vi "nav_test.vi"() -> ()   [LabVIEW 2009]
uses:
  Seagle_2010_v2.0 - rewrite.llb/GPGLL data.ctl
  Seagle_2010_v2.0 - rewrite.llb/GPVTG data.ctl
  Seagle_2010_v2.0 - rewrite.llb/GPGSA data.ctl
  Seagle_2010_v2.0 - rewrite.llb/GPGSV data.ctl
  Seagle_2010_v2.0 - rewrite.llb/GPRMC data.ctl
  Seagle_2010_v2.0 - rewrite.llb/GPSINS output.ctl
  <vilib>/Instr/_visa.llb/VISA Configure Serial Port (Instr).vi
  Seagle_2010_v2.0 - rewrite.llb/GPS_Data_Global_Var.vi
panel:
  in  "Tab Control":enum32{"Motors", "GPS", "Compass", "COM"}(tab)
  in  "Percent Throttle":dbl(slide)=1.0 scale=0.0..1.0
  in  "scale turn":dbl(slide)=0.23 scale=0.0..1.0
  out "Effective Gain":dbl
  in  "Forward Gain":dbl=0.5
  in  "Exponential":dbl=0.7
  in  "kd":dbl
  in  "Deadband (Deg)":dbl=5.0
  out "Left Motor (V)":dbl=1.8685682059795314
  out "Right Motor (V)":dbl=3.166227290921547
  out "GPS Status":T1={"GPS Connected"=TRUE, "GPS Connect Status"="Connected at 9600"}
  in  "Reset\nComp?":bool
  out "GPS cluster":T2={"Easting "=166021.4430837002, "Northing"=0.0, "Horizontal Speed (m/s)"=0.0, "Heading (degrees)"=0.0, "Pitch (degrees)"=0.0, "Roll (degrees)"=0.0, "IMU Alignment"="", "Hardware Status"="Insuff OBS", "Solution (Novatel)"="No Pos Info", "Altitude (m)"=-6378054.200000763, "Vertical Speed (m/s)"=0.0, "Seconds"=1541650, "Standard Deviation (Lat, m)"=0.0, "Standard Deviation (Long, m)"=0.0} {"Northing" format="%#.2f"; "Easting" format="%#.2f"}
  out "GPS Online":bool
  out "Updated Data?":bool
  in  "GPS Waypoint File Path":path=path "C:/Documents and Settings/Seagle09/Desktop/final waypoints/final.txt"
  out "GPS Data":T3={"Easting"=166021.4430837002, "Northing"=0.0, "Status"="No Pos Info"} {"Easting" format="%#.10f"; "Northing" format="%#.10f"}
  in  "Enum":T4(ring)=enum."New Novatel"
  in  "Reset GPS Wypts?":bool
  in  "GPS Drive Point":cluster{"Easting":ext, "Northing":ext}={"Easting"=393714.5212, "Northing"=4073667.644} {"Northing" format="%#_10f"; "Easting" format="%#_10f"}
  out "GPS Error":errorcluster={"status"=FALSE, "code"=1073676294, "source"="VISA Read in Novatel_get_data.vi->Read Novatel_2.0.vi->Seagle.vi"}
  out "Waypoints \nComplete":bool
  out "Comp Time":u32=1520
  in  "Compass Enable":bool=TRUE
  out "Compass Error":errorcluster={"status"=FALSE, "code"=1073676294, "source"="VISA Read in Compass Parse.vi->Seagle.vi"}
  out "Compass Data":T5={"Heading (deg)"=8.7, "Pitch (deg)"=0.8, "Roll (deg)"=1.6}
  out "Comp Online?":bool=TRUE
  in  "GPS & Compass Com Ports":T6={"Comp Com"="COM7", "GPS Com"="COM8"}
  in  "Tab Control 2":T7(tab)
  out "Satellites\nUsed":dbl
  out "Satellite Constellation":cluster{sgl[], sgl[]}[](graph)
  out "UTC Date":string
  out "?":enum16{"Meters", "Unrecognized"}(ring)
  out "Altitude":sgl
  out "DGPS Age":sgl
  out "Satellites\nin View":dbl
  out "Solution":T8(ring)
  out "UTC Seconds":sgl
  out "UTC Minutes":i32
  out "UTC Hours":i32
  out "North/South":enum16{"North", "South"}(ring)
  out "Lat Minutes":sgl
  out "Degrees":i32
  out "East/West":enum16{"East", "West"}(ring)
  out "Minutes":sgl
  out "Deg.":i32
  out "Serial Error":errorcluster
  out "GPRMC Data":T9
  out "GPGSV Data":T10
  out "GPGSA Data":T11
  out "GPVTG\nData":T12
  out "GPGLL\nData":T13
  out "Satellite Constellation Plot":cluster{sgl[], sgl[]}[](graph)
  in  "parallax com port":refnum<visa-resource-name>="COM10"
  in  "Parallax baud rate":u32=2400
  in  "stop":bool
  # "Longitude"
  # "UTC Time"
  # "Lattitude"
  # ":"
  # ":"
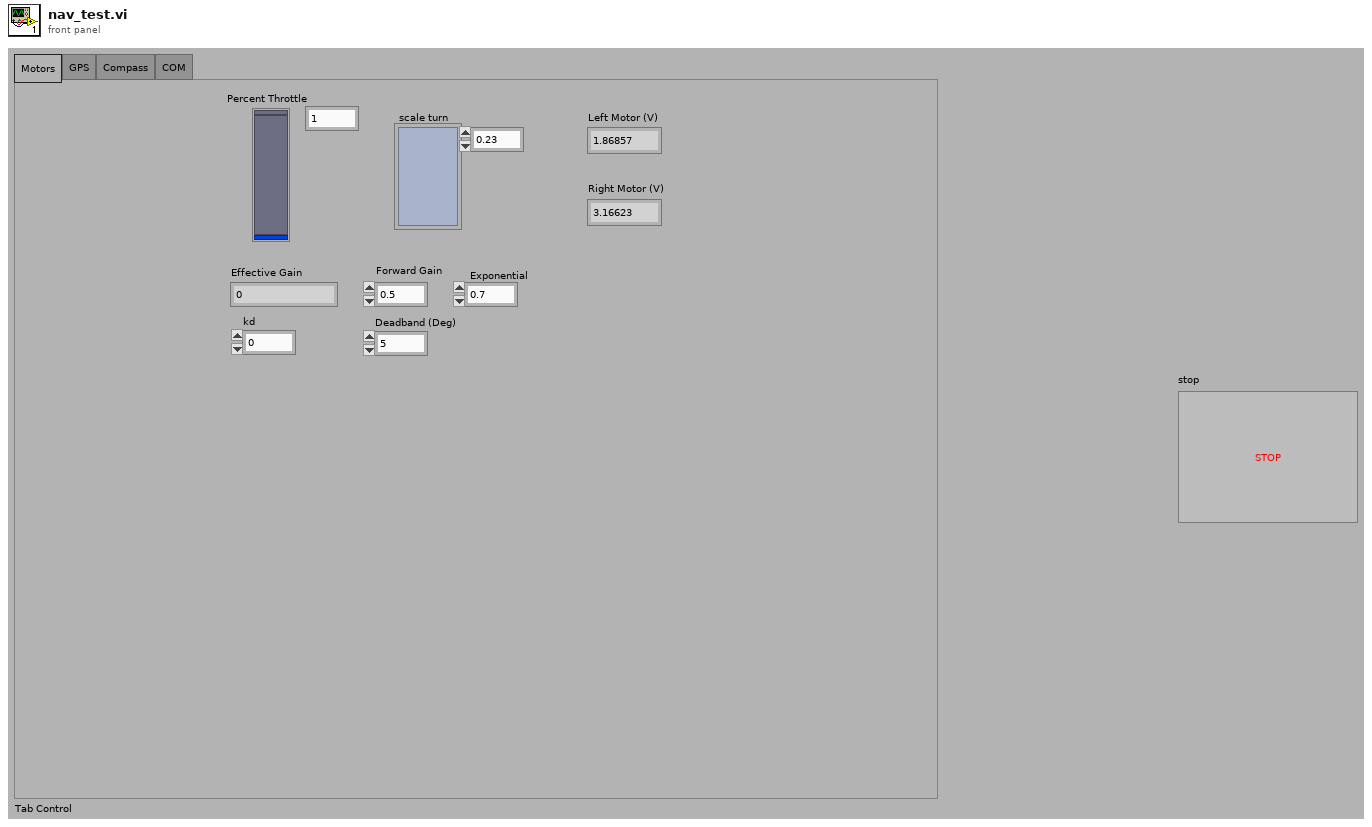
[diagram p1: front panel]
types:
  T1 = cluster{"GPS Connected":bool, "GPS Connect Status":string}
  T2 = typedef "GPSINS output.ctl" = cluster{"Easting ":dbl, "Northing":dbl, "Horizontal Speed (m/s)":dbl, "Heading (degrees)":dbl, "Pitch (degrees)":dbl, "Roll (degrees)":dbl, "IMU Alignment":string, "Hardware Status":string, "Solution (Novatel)":string, "Altitude (m)":dbl, "Vertical Speed (m/s)":dbl, "Seconds":u32, "Standard Deviation (Lat, m)":dbl, "Standard Deviation (Long, m)":dbl}
  T3 = cluster{"Easting":dbl, "Northing":dbl, "Status":string}
  T4 = enum16{"Ublox", "No GPS", "New Novatel", "Old Novatel"}
  T5 = cluster{"Heading (deg)":dbl, "Pitch (deg)":dbl, "Roll (deg)":dbl}
  T6 = cluster{"Comp Com":refnum<visa-resource-name>, "GPS Com":refnum<visa-resource-name>}
  T7 = enum32{"Main Display", "Controls", "GPRMC", "GPGSV", "GPGSA", "GPGGA", "GPVTG", "GPGLL", "Satellites"}
  T8 = enum16{"Invalid", "Valid SPS", "Valid DGPS", "Valid PPS"}
  T9 = typedef "GPRMC data.ctl" = cluster{"UTC Hours":i32, "UTC Minutes":i32, "UTC Seconds":sgl, "Solution status":enum16{"Valid", "Invalid"}, "Lat Degrees":i32, "Lat Minutes":sgl, "North/South":enum16{"North", "South"}, "Long. Degrees":i32, "Long. Minutes":sgl, "East/West":enum16{"East", "West"}, "Speed Over\nGround":sgl, "Course Over\nGround":sgl, "UTC Date":string, "Magnetic \nVariation\n(deg)":sgl, "East/West":enum16{"East", "West"}, "Data\nReceived":bool}
  T10 = typedef "GPGSV data.ctl" = cluster{"Number of\nMessages":dbl, "Sequence\nNumber":dbl, "Satellites\nin View":dbl, "Sattelite Info":cluster{" ID":dbl, "Elev.":dbl, "Azi.":dbl, "SNR":dbl}[], "Data Received":bool}
  T11 = typedef "GPGSA data.ctl" = cluster{"GPS Mode 1(a)":enum16{"Auto 2D/3D", "Forced 2D/3D"}, "GPS Mode 1(b)":enum16{"No Fix", "2-D", "3-D"}, "Sat 1":i32, "Sat 2":i32, "Sat 3":i32, "Sat 4":i32, "Sat 5":i32, "Sat 6":i32, "Sat 7":i32, "Sat 8":i32, "Sat 9":i32, "Sat 10":i32, "Sat 11":i32, "Sat 12":i32, "PDOP":sgl, "HDOP":sgl, "VDOP":sgl, "Data\nReceived":bool}
  T12 = typedef "GPVTG data.ctl" = cluster{"Track made Good":sgl, enum16{"True Heading", "Magnetic heading"}, "TMG":sgl, enum16{"True Heading", "Magnetic heading"}, "Speed over Gnd":sgl, enum16{"Km/hr", "Knots"}, "Speed over Gnd":sgl, enum16{"Km/hr", "Knots"}, "Data\n Received":bool}
  T13 = typedef "GPGLL data.ctl" = cluster{"Lat Degrees":i32, "Lat Minutes":sgl, "North/South":enum16{"North", "South"}, "Long. Degrees":i32, "Long. Minutes":sgl, "East/West":enum16{"East", "West"}, "UTC Hours":i32, "UTC Minutes":i32, "UTC Seconds":sgl, "position":enum16{"Valid", "Invalid"}, "Data\nReceived":bool}
  T14 = enum16{"VT Challenge 1", "VT Challenge 2", "IGVC"}
  T15 = cluster{"Servo Position 0":i32, "Servo Position 1":i32, "Servo Position 2":i32, "Servo Position 3":i32, "Servo Position 4":i32, "Servo Position 5":i32, "Servo Position 6":i32, "Servo Position 7":i32, "Servo Position 8":i32, "Servo Position 9":i32, "Servo Position 10":i32, "Servo Position 11":i32, "Servo Position 12":i32, "Servo Position 13":i32, "Servo Position 14":i32, "Servo Position 15":i32}
  T16 = cluster{"Waypoint num":dbl, "Eastint (m)":ext, "Northing (m)":ext}[]
  T17 = cluster{"Current Waypoint":i32, "Number of Waypoints":i32, "Dist to wapoint (m)":dbl, "Desired Direction (deg)":dbl}
  T18 = cluster{"Dist to wapoint (m)":dbl, "Desired Direction (deg)":dbl}
  T19 = cluster{"Easting":dbl, "Northing":dbl, "Sol'n":string}
  T20 = typedef "NMEA_Data.ctl" = cluster{"GPGSA Data":cluster{"GPS Mode 1(a)":enum16{"Auto 2D/3D", "Forced 2D/3D"}, "GPS Mode 1(b)":enum16{"No Fix", "2-D", "3-D"}, "Sattllite used 1":i32, "Sattllite used 2":i32, "Sattllite used 3":i32, "Sattllite used 4":i32, "Sattllite used 5":i32, "Sattllite used 6":i32, "Sattllite used 7":i32, "Sattllite used 8":i32, "Sattllite used 9":i32, "Sattllite used 10":i32, "Sattllite used 11":i32, "Sattllite used 12":i32, "PDOP":sgl, "HDOP":sgl, "VDOP":sgl, "Data Received":bool}, "GPGGA\nData":T21, "GPRMC Data":cluster{"UTC Hours":i32, "UTC Minutes":i32, "UTC Seconds":sgl, enum16{"Valid", "Invalid"}, "Lat Degrees":i32, "Lat Minutes":sgl, "North/South":enum16{"North", "South"}, "Long. Degrees":i32, "Long. Minutes":sgl, "East/West":enum16{"East", "West"}, "Speed Over\nGround":sgl, "Course Over\nGround":sgl, "UTC Date":string, "Magnetic Variation\n(deg)":sgl, "East/West":enum16{"East", "West"}, "Data Received":bool}, "GPGLL\nData":cluster{"Lat Degrees":i32, "Lat Minutes":sgl, "North/South":enum16{"North", "South"}, "Long. Degrees":i32, "Long. Minutes":sgl, "East/West":enum16{"East", "West"}, "UTC Hours":i32, "UTC Minutes":i32, "UTC Seconds":sgl, enum16{"Valid", "Invalid"}, "Data Received":bool}, "GPGSV\nData":cluster{"Number of\nMessages":dbl, "Sequence\nNumber":dbl, "Satellites\nin View":dbl, "Sattelite Info":cluster{" ID":dbl, "Elev.":dbl, "Azi.":dbl, "SNR":dbl}[], "Data Received":bool}, "GPVTG\nData":cluster{"Float":sgl, enum16{"True Heading", "Magnetic heading"}, "Float":sgl, enum16{"True Heading", "Magnetic heading"}, "Float":sgl, enum16{"Km/hr", "Knots"}, "Float":sgl, enum16{"Km/hr", "Knots"}, "Data Received":bool}, "GPGST Data":T22}
  T21 = typedef "GPGGA data.ctl" = cluster{"UTC Hours":i32, "UTC Minutes":i32, "UTC Seconds":sgl, "Lat Degrees":i32, "Lat Minutes":sgl, "North/South":enum16{"North", "South"}, "Long. Degrees":i32, "Long. Minutes":sgl, "East/West":enum16{"East", "West"}, "Status":enum16{"Invalid", "Valid SPS", "Valid DGPS", "Valid PPS"}, "Sats. Used":i32, "HDOP":sgl, "Altitude":sgl, "Altitude Units":enum16{"Meters", "Unrecognized"}, "Geoid Separation":sgl, "Geoid Seperation Units":enum16{"Meters", "Unrecognized"}, "DGPS Age":sgl, "DGPS Station ID":i32, "Data\nReceived":bool, "Status string":string}
  T22 = typedef "GPGST data.ctl" = cluster{"UTC Hours":i32, "UTC Minutes":i32, "UTC Seconds":sgl, "Total RMS \nStandard Deviation":sgl, "St Dev of Semi-Major\naxis of Error Elipse":sgl, "St Dev of Semi-Minor\naxis of Error Elipse":sgl, "Orientation of Semi-Major\naxis of Error Elipse (True North deg)":sgl, "St Dev Lat (m)":sgl, "St Dev Long (m)":sgl, "St Dev Alt (m)":sgl, "Data Received":bool}
  T23 = cluster{"GPS Mode 1(a)":enum16{"Auto 2D/3D", "Forced 2D/3D"}, "GPS Mode 1(b)":enum16{"No Fix", "2-D", "3-D"}, "Sattllite used 1":i32, "Sattllite used 2":i32, "Sattllite used 3":i32, "Sattllite used 4":i32, "Sattllite used 5":i32, "Sattllite used 6":i32, "Sattllite used 7":i32, "Sattllite used 8":i32, "Sattllite used 9":i32, "Sattllite used 10":i32, "Sattllite used 11":i32, "Sattllite used 12":i32, "PDOP":sgl, "HDOP":sgl, "VDOP":sgl, "Data Received":bool}
  T24 = cluster{"UTC Hours":i32, "UTC Minutes":i32, "UTC Seconds":sgl, enum16{"Valid", "Invalid"}, "Lat Degrees":i32, "Lat Minutes":sgl, "North/South":enum16{"North", "South"}, "Long. Degrees":i32, "Long. Minutes":sgl, "East/West":enum16{"East", "West"}, "Speed Over\nGround":sgl, "Course Over\nGround":sgl, "UTC Date":string, "Magnetic Variation\n(deg)":sgl, "East/West":enum16{"East", "West"}, "Data Received":bool}
  T25 = cluster{"Lat Degrees":i32, "Lat Minutes":sgl, "North/South":enum16{"North", "South"}, "Long. Degrees":i32, "Long. Minutes":sgl, "East/West":enum16{"East", "West"}, "UTC Hours":i32, "UTC Minutes":i32, "UTC Seconds":sgl, enum16{"Valid", "Invalid"}, "Data Received":bool}
  T26 = cluster{"Number of\nMessages":dbl, "Sequence\nNumber":dbl, "Satellites\nin View":dbl, "Sattelite Info":cluster{" ID":dbl, "Elev.":dbl, "Azi.":dbl, "SNR":dbl}[], "Data Received":bool}
  T27 = cluster{"Float":sgl, enum16{"True Heading", "Magnetic heading"}, "Float":sgl, enum16{"True Heading", "Magnetic heading"}, "Float":sgl, enum16{"Km/hr", "Knots"}, "Float":sgl, enum16{"Km/hr", "Knots"}, "Data Received":bool}
  T28 = typedef "GPSINS outputb.ctl" = cluster{"Easting ":dbl, "Northing":dbl, "Horizontal Speed (m/s)":dbl, "Heading (degrees)":dbl, "Pitch (degrees)":dbl, "Roll (degrees)":dbl, "IMU Alignment":string, "Hardware Status":string, "Solution (Novatel)":string, "Altitude (m)":dbl, "Vertical Speed (m/s)":dbl, "Seconds":u32, "Standard Deviation (Lat, m)":dbl, "Standard Deviation (Long, m)":dbl}
  T29 = cluster{"Solution Status":u32, "Latitude (deg)":dbl, "Longitude (deg)":dbl, "Height (m)":dbl, "Latitude Std Dev (m)":sgl, "Longitude Std Dev (m)":sgl, "Height Std Dev (m)":sgl, "Position Type":u32, "Datum ID Number":u32}
  T30 = cluster{"Heading":dbl, "Pitch":dbl, "Roll":dbl, "Temp":dbl, "Check Sum":string, "Status":bool}
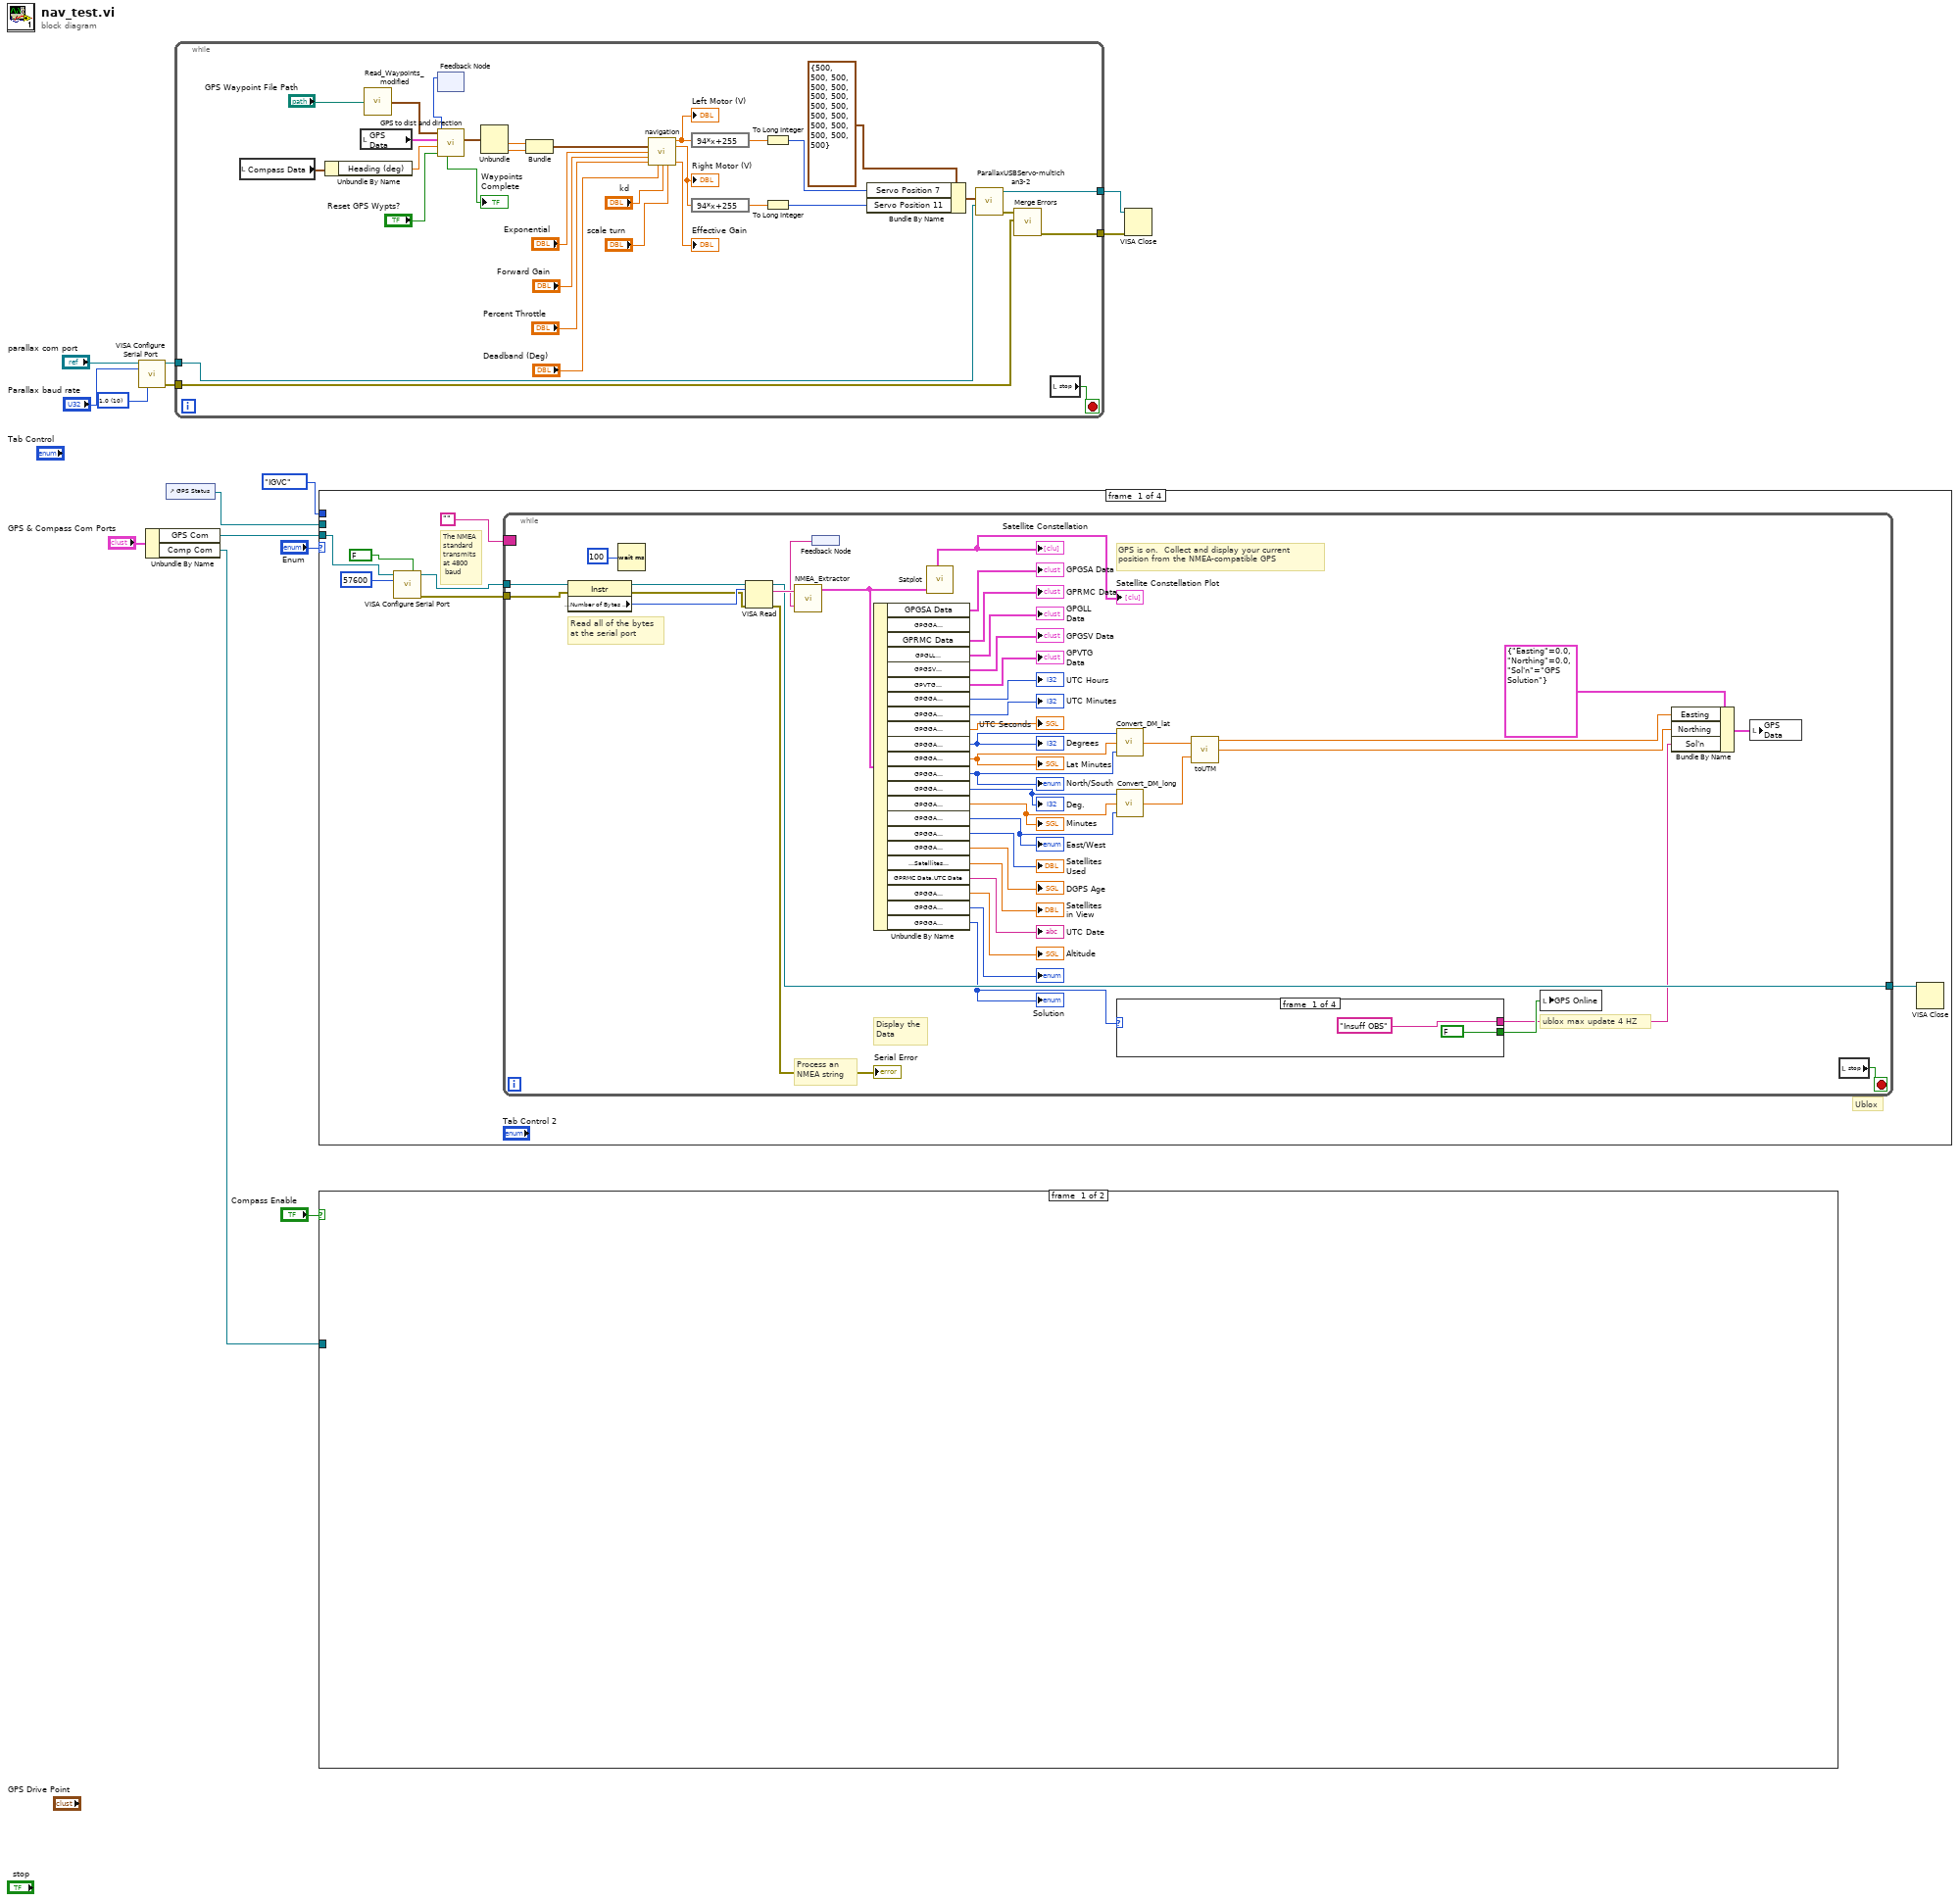
[diagram p0: block diagram]
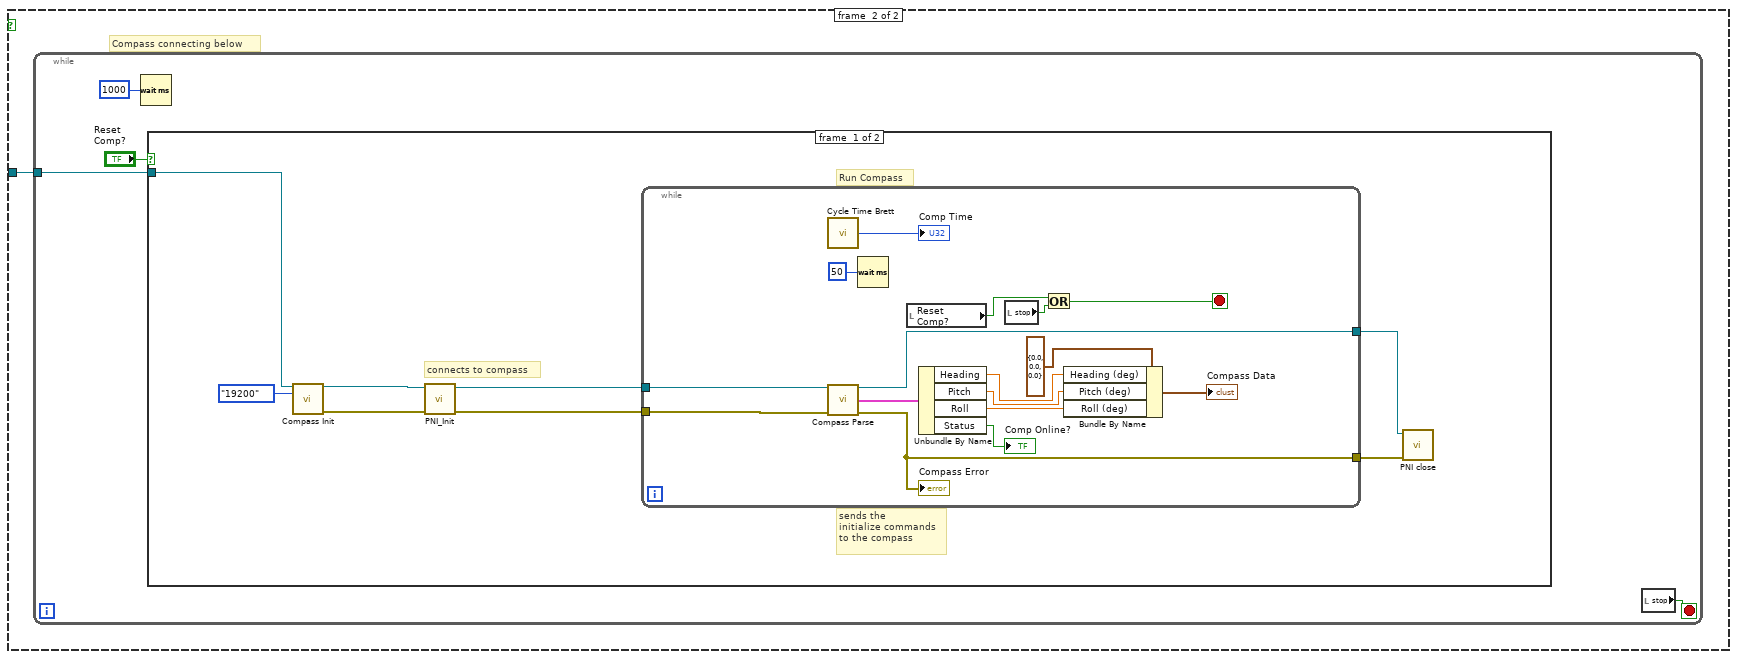
[diagram p2: hidden frame]
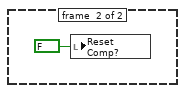
[diagram p3: hidden frame]
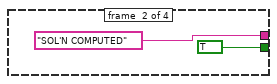
[diagram p4: hidden frame]
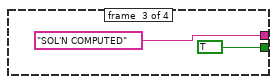
[diagram p5: hidden frame]
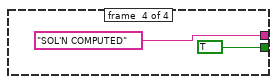
[diagram p6: hidden frame]
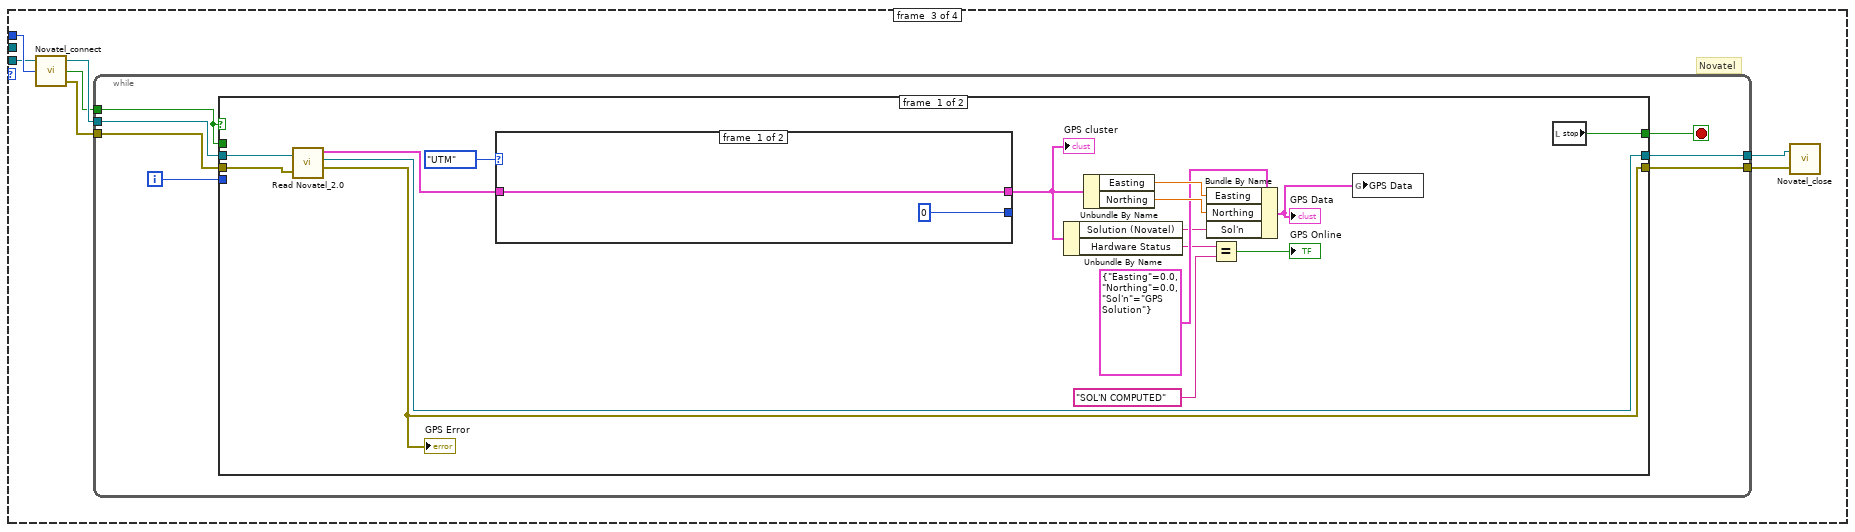
[diagram p8: hidden frame]
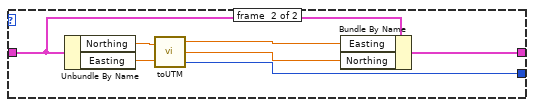
[diagram p9: hidden frame]
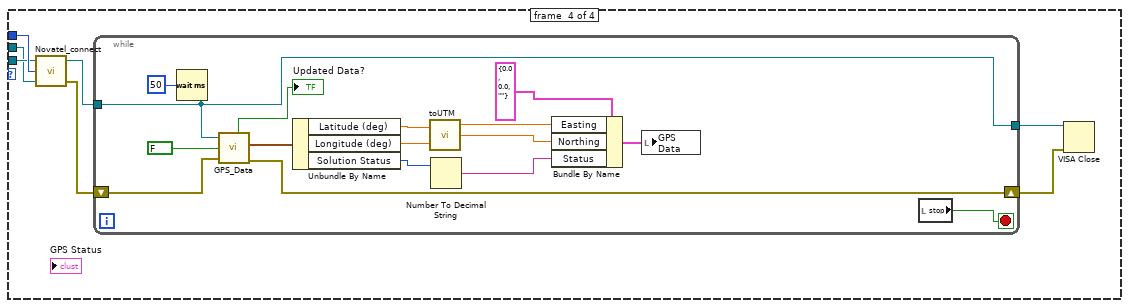
[diagram p11: hidden frame]
diagram:
  w8 = u16 10 items=["1.0"=10, "1.5"=15, "2.0"=20] ("stop bits (10: 1 bit)")
  n1 = call-poly "VISA Configure Serial Port"("VISA resource name"="parallax com port", "baud rate (9600)"="Parallax baud rate", "stop bits (10: 1 bit)"=w8) -> ("VISA resource name out"=w5:refnum<visa-resource-name>, "error out"=w4:errorcluster)  [unwired: 4 in, 7 out]
  n2 = Unbundle By Name("GPS & Compass Com Ports") -> ("GPS Com"=w12:refnum<visa-resource-name>, "Comp Com"=w13:refnum<visa-resource-name>)
  n3 = control-ref of="GPS Status"() -> (w1:refnum<vi>)
  n4 = while {
    tunnel: w5 -> [w19]
    tunnel: w4 -> [w17]
    tunnel: [w16] -> w3
    tunnel: [w15] -> w2
    stop <- w41 stop-if-true
    n5 = local read "Compass Data"() -> (w39:T5)
    n6 = Unbundle By Name(w39) -> ("Heading (deg)"=w38:dbl)
    n7 = local read "GPS Data"() -> (w33:T3)
    n8 = call "Read_Waypoints_modified.vi"("Waypoint File Path:"="GPS Waypoint File Path") -> ("Waypoints"=w37:T16)
    n9 = feedback #1() -> (w36:i32)  [unwired: 1 in]
    n10 = call "GPS to dist and direction.vi"("Current Waypoint (in)"=w36, "Reset Wypts?"="Reset GPS Wypts?", "Current Heading (deg)"=w38, "GPS Data IN"=w33, "Waypoints"=w37) -> ("Waypoint info"=w32:T17, "Current Waypoint (out)"=w34:i32, "Waypoints \nComplete"=→"Waypoints \nComplete":bool)  [unwired: 4 out]
    n11 = Unbundle(w32) -> ("Dist to wapoint (m)"=w31:dbl, "Desired Direction (deg)"=w30:dbl)  [unwired: 2 out]
    n12 = Bundle("Dist to wapoint (m)"=w31, "Desired Direction (deg)"=w30) -> (w29:T18)  [unwired: 1 in]
    n13 = call "navigation.vi"("Drive point"=w29, "Exponent"="Exponential", "Forward Gain"="Forward Gain", "Percent Throttle"="Percent Throttle", "Deadband"="Deadband (Deg)", "kd"="kd", "scale turn"="scale turn") -> ("Left Motor (v)"=w28:dbl, "Right Motor (v)"=w27:dbl, "Effective Gain Range (m)"=→"Effective Gain":dbl)  [unwired: 5 in, 1 out]
    "Left Motor (V)" <- w28
    "Right Motor (V)" <- w27
    n14 = expression code="94*x+255"(w28) -> (w25:dbl)
    n15 = expression code="94*x+255"(w27) -> (w24:dbl)
    n16 = To Long Integer(number=w25) -> (32bit integer=w22:i32)
    n17 = To Long Integer(number=w24) -> (32bit integer=w23:i32)
    n18 = Bundle By Name(cluster=T15 {"Servo Position 0"=500, "Servo Position 1"=500, "Servo Position 2"=500, "Servo Position 3"=500, "Servo Position 4"=500, "Servo Position 5"=500, "Servo Position 6"=500, "Servo Position 7"=500, "Servo Position 8"=500, "Servo Position 9"=500, "Servo Position 10"=500, "Servo Position 11"=500, "Servo Position 12"=500, "Servo Position 13"=500, "Servo Position 14"=500, "Servo Position 15"=500} ("Servo Cluster"), "Servo Position 7"=w22, "Servo Position 11"=w23) -> (w20:T15)
    n19 = call "ParallaxUSBServo-multichan3-2.vi"("VISA resource"=w19, "Servo Cluster"=w20) -> ("error out"=w18:errorcluster, "VISA resource"=w16:refnum<visa-resource-name>)  [unwired: 8 out]
    n20 = call <vilib>:"Merge Errors.vi"("error in 2 (no error)"=w17, "error in 1 (no error)"=w18) -> ("error out"=w15:errorcluster)  [unwired: 2 in, 3 out]
    n21 = local read "stop"() -> (w41:bool)
  }
  n22 = case shown="\"Old Novatel\"" "Enum" {
    tunnel: w1 -> [_ _ _ w149]
    tunnel: T14."IGVC" ("Configuration Type") -> [_ _ w108 w151]
    tunnel: w12 -> [w49 _ w107 w150]
    frame #0 {
      # "The NMEA\nstandard \ntransmits\nat 4800\n baud"
      # "Ublox"
      n23 = call-poly "VISA Configure Serial Port"("VISA resource name"=w49, "Enable Termination\nChar (T)"=FALSE ("Enable Termination\nChar (T)"), "baud rate (9600)"=u32 57600) -> ("VISA resource name out"=w51:refnum<visa-resource-name>, "error out"=w52:errorcluster)  [unwired: 4 in, 7 out]
      n24 = while {
        tunnel: w51 -> [w98]
        tunnel: w52 -> [w94]
        tunnel: [w76] -> w55
        border: "" ("Empty String Constant") -> [_]
        stop <- w63 stop-if-true
        # "ublox max update 4 HZ"
        # "GPS is on.  Collect and display your current\nposition from the NMEA-compatible GPS"
        # "Display the\nData"
        # "Process an \nNMEA string"
        # "Read all of the bytes\nat the serial port"
        n25 = property on="Property Node" class="Instr"(reference=w98, error in=w94) -> (reference out=w97:refnum<visa-resource-name>, error out=w95:errorcluster, "Serial Settings:Number of Bytes at Serial Port"=w96:u32)
        n26 = Wait (ms)(milliseconds to wait=u32 100 ("millisecond multiple")) -> ()  [unwired: 1 out]
        n27 = VISA Read(VISA resource name=w97, byte count=w96, error in (no error)=w95) -> (VISA resource name out=w76:refnum<visa-resource-name>, read buffer=w93:string, error out=→"Serial Error":errorcluster)  [unwired: 1 out]
        n28 = feedback #2() -> (w92:string)
        n29 = call "NMEA_Extractor.vi"("New Data"=w93, "Previous Data\n(none = default)"=w92) -> ("NMEA Data"=w77:T20, "Leftover Data"=w91:string)  [unwired: 1 out]
        n30 = Unbundle By Name(w77) -> ("GPGSA Data"=→"GPGSA Data":T23, "GPRMC Data"=→"GPRMC Data":T24, "GPGLL\nData"=→"GPGLL\nData":T25, "GPGSV\nData"=→"GPGSV Data":T26, "GPVTG\nData"=→"GPVTG\nData":T27, "GPGGA\nData.UTC Hours"=→"UTC Hours":i32, "GPGGA\nData.UTC Minutes"=→"UTC Minutes":i32, "GPGGA\nData.UTC Seconds"=→"UTC Seconds":sgl, "GPGGA\nData.Lat Degrees"=w74:i32, "GPGGA\nData.Lat Minutes"=w69:sgl, "GPGGA\nData.North/South"=w73:enum16{"North", "South"}, "GPGGA\nData.Long. Degrees"=w71:i32, "GPGGA\nData.Long. Minutes"=w70:sgl, "GPGGA\nData.East/West"=w72:enum16{"East", "West"}, "GPGGA\nData.Sats. Used"=→"Satellites\nUsed":i32, "GPGGA\nData.DGPS Age"=→"DGPS Age":sgl, "GPGSV\nData.Satellites\nin View"=→"Satellites\nin View":dbl, "GPRMC Data.UTC Date"=→"UTC Date":string, "GPGGA\nData.Altitude"=→"Altitude":sgl, "GPGGA\nData.Altitude Units"=→"?":enum16{"Meters", "Unrecognized"}, "GPGGA\nData.Status"=w62:T8)  [unwired: 1 out]
        "Deg." <- w71
        "Minutes" <- w70
        "East/West" <- w72
        "North/South" <- w73
        "Lat Minutes" <- w69
        "Degrees" <- w74
        "Solution" <- w62
        n31 = call "Satplot.vi"("NMEA Data"=w77) -> ("Array"=→"Satellite Constellation Plot" →"Satellite Constellation":cluster{sgl[], sgl[]}[])  [unwired: 4 out]
        n32 = call "Convert_DM_lat.vi"("North/South"=w73, "Lat Minutes"=w69, "Lat Degrees"=w74) -> ("Numeric"=w68:sgl)
        n33 = call "Convert_DM_long.vi"("East/West"=w72, "Long. Minutes"=w70, "Long. Degrees"=w71) -> ("Numeric"=w67:sgl)
        n34 = case shown="\"Valid SPS\"" w62 {
          tunnel: [FALSE TRUE TRUE TRUE] -> w61
          tunnel: ["Insuff OBS" ("IMU Alignment") "SOL'N COMPUTED" ("IMU Alignment") "SOL'N COMPUTED" ("IMU Alignment") "SOL'N COMPUTED" ("IMU Alignment")] -> w57
          frame #0 {
          }
          frame #1 {
          }
          frame #2 {
          }
          frame #3 {
          }
        }
        n35 = call "toUTM.vi"("Lat (dec deg)"=w68, "Long (dec deg)"=w67) -> ("Easting (m)"=w59:dbl, "Northing (m)"=w58:dbl)  [unwired: 1 out]
        n36 = local write "GPS Online"(w61) -> ()
        n37 = Bundle By Name(cluster=T19 {"Easting"=0.0, "Northing"=0.0, "Sol'n"="GPS Solution"}, "Easting"=w59, "Northing"=w58, "Sol'n"=w57) -> (w56:T19)
        n38 = local write "GPS Data"(w56) -> ()
        n39 = local read "stop"() -> (w63:bool)
      }
      n40 = VISA Close(VISA resource name=w55) -> ()  [unwired: 1 in, 1 out]
    }
    frame #1 {
    }
    frame #2 {
      # "Novatel"
      n41 = call "Novatel_connect.vi"("Configuration Type"=w108, "VISA resource name"=w107) -> ("error out"=w112:errorcluster, "Cancel?"=w111:bool, "dup VISA resource name"=w113:refnum<visa-resource-name>)  [unwired: 1 in]
      n42 = while {
        tunnel: w113 -> [w120]
        tunnel: w112 -> [w119]
        tunnel: [w118] -> w110
        tunnel: [w117] -> w109
        tunnel: w111 -> [w115]
        i -> [w114]
        stop <- w116 stop-if-true
        n43 = case shown="False" w115 {
          tunnel: w120 -> [w136 w148]
          tunnel: w119 -> [w135 w147]
          tunnel: [w134 w148] -> w118
          tunnel: [w130 w147] -> w117
          tunnel: [w131 w146] -> w116
          tunnel: w115 -> [_ w146]
          tunnel: w114 -> [_ _]
          frame #0 {
            n44 = call "Read Novatel_2.0.vi"("VISA resource name"=w136, "error in (no error)"=w135) -> ("IMU/GPS data"=w132:T28, "dup VISA resource name"=w134:refnum<visa-resource-name>, "error out"=w130:errorcluster)  [unwired: 1 out]
            "GPS Error" <- w130
            n45 = case shown="\"UTM\"" enum16{"LAT/LONG", "UTM"}."UTM" ("Position Units") {
              tunnel: w132 -> [w137 w143]
              tunnel: [u8 0 ("Zone") w140] -> _
              tunnel: [w137 w139] -> w127
              frame #0 {
              }
              frame #1 {
                n46 = Unbundle By Name(w143) -> ("Northing"=w145:dbl, "Easting"=w144:dbl)
                n47 = call "toUTM.vi"("Lat (dec deg)"=w145, "Long (dec deg)"=w144) -> ("Easting (m)"=w142:dbl, "Northing (m)"=w141:dbl, "Zone"=w140:u8)
                n48 = Bundle By Name(cluster=w143, "Easting"=w142, "Northing"=w141) -> (w139:T28)
              }
            }
            "GPS cluster" <- w127
            n49 = Unbundle By Name(w127) -> ("Solution (Novatel)"=w123:string, "Hardware Status"=w122:string)
            n50 = Unbundle By Name(w127) -> ("Easting"=w126:dbl, "Northing"=w125:dbl)
            n51 = Bundle By Name(cluster=T19 {"Easting"=0.0, "Northing"=0.0, "Sol'n"="GPS Solution"}, "Easting"=w126, "Northing"=w125, "Sol'n"=w123) -> (w121:T19)
            "GPS Data" <- w121
            n52 = Equal?(x=w122, y="SOL'N COMPUTED" ("IMU Alignment")) -> (x = y?=→"GPS Online":bool)
            n53 = global write "GPS_Data_Global_Var.vi" "GPS Data"(w121) -> ()
            n54 = local read "stop"() -> (w131:bool)
          }
          frame #1 {
          }
        }
      }
      n55 = call "Novatel_close.vi"("error in"=w109, "dup VISA resource name"=w110) -> ()  [unwired: 1 out]
    }
    frame #3 {
      n56 = call "Novatel_connect.vi"("GPS Connection Status"=w149, "Configuration Type"=w151, "VISA resource name"=w150) -> ("error out"=w152:errorcluster, "dup VISA resource name"=w153:refnum<visa-resource-name>)  [unwired: 1 out]
      n57 = while {
        tunnel: w153 -> [w168]
        tunnel: [w168] -> w154
        shift-right: [w170] -> w155
        shift-left: w152 -> [w167]
        stop <- w165 stop-if-true
        n58 = Wait (ms)(milliseconds to wait=u32 50) -> ()  [unwired: 1 out]
        n59 = call "GPS_Data.vi"("error in (no error)"=w167, "Use CRC?"=FALSE, "VISA resource name"=w168) -> ("error out"=w170:errorcluster, "BestPos Out"=w169:T29, "Updated Data?"=→"Updated Data?":bool)  [unwired: 3 out]
        n60 = Unbundle By Name(w169) -> ("Latitude (deg)"=w163:dbl, "Longitude (deg)"=w162:dbl, "Solution Status"=w158:u32)
        n61 = call "toUTM.vi"("Lat (dec deg)"=w163, "Long (dec deg)"=w162) -> ("Easting (m)"=w161:dbl, "Northing (m)"=w160:dbl)  [unwired: 1 out]
        n62 = Number To Decimal String(number=w158) -> (decimal integer string=w157:string)  [unwired: 1 out]
        n63 = Bundle By Name(cluster=T3 {"Easting"=0.0, "Northing"=0.0, "Status"=""} ("GPS Data"), "Easting"=w161, "Northing"=w160, "Status"=w157) -> (w159:T3)
        n64 = local write "GPS Data"(w159) -> ()
        n65 = local read "stop"() -> (w165:bool)
      }
      n66 = VISA Close(VISA resource name=w154, error in (no error)=w155) -> ()  [unwired: 1 out]
    }
  }
  n67 = case shown="True" "Compass Enable" {
    tunnel: w13 -> [_ w172]
    frame #0 {
    }
    frame #1 {
      # "Compass connecting below"
      n68 = while {
        tunnel: w172 -> [w173]
        stop <- w175 stop-if-true
        n69 = Wait (ms)(milliseconds to wait=u32 1000) -> ()  [unwired: 1 out]
        n70 = case shown="False" "Reset\nComp?" {
          tunnel: w173 -> [w181 _]
          frame #0 {
            # "connects to compass"
            # "sends the \ninitialize commands\nto the compass"
            # "Run Compass"
            n71 = call "Compass Init.vi"("VISA resource name"=w181, "Baud Rate"=enum16{"9600", "19200"}."19200") -> ("duplicate VISA resource name"=w179:refnum<visa-resource-name>, "error out"=w178:errorcluster)  [unwired: 2 in, 10 out]
            n72 = call "PNI_Init.vi"("error in (no error)"=w178, "VISA resource name"=w179) -> ("error out"=w177:errorcluster, "VISA resource name out"=w180:refnum<visa-resource-name>)  [unwired: 1 in, 7 out]
            n73 = while {
              tunnel: [w200] -> w184
              tunnel: [w199] -> w183
              tunnel: w180 -> [w190]
              tunnel: w177 -> [w186]
              stop <- w189 stop-if-true
              n74 = call "Cycle Time Brett.vi"() -> ("Cycle Time"=→"Comp Time":u32)
              n75 = call "Compass Parse.vi"("VISA resource name"=w190, "error in (no error)"=w186) -> ("Dup VISA resource name"=w200:refnum<visa-resource-name>, "Compass Data (num)"=w197:T30, "error out"=w199:errorcluster)  [unwired: 11 out]
              "Compass Error" <- w199
              n76 = Wait (ms)(milliseconds to wait=u32 50) -> ()  [unwired: 1 out]
              n77 = local read "Reset\nComp?"() -> (w188:bool)
              n78 = Unbundle By Name(w197) -> ("Heading"=w195:dbl, "Pitch"=w194:dbl, "Roll"=w193:dbl, "Status"=→"Comp Online?":bool)
              n79 = local read "stop"() -> (w185:bool)
              n80 = Or(x=w188, y=w185) -> (x .or. y?=w189:bool)
              n81 = Bundle By Name(cluster=T5 {"Heading (deg)"=0.0, "Pitch (deg)"=0.0, "Roll (deg)"=0.0} ("Compass Data OUT"), "Heading (deg)"=w195, "Pitch (deg)"=w194, "Roll (deg)"=w193) -> (→"Compass Data":T5)
            }
            n82 = call "PNI close.vi"("error in (no error)"=w183, "VISA resource name"=w184) -> ()  [unwired: 10 out]
          }
          frame #1 {
            n83 = local write "Reset\nComp?"(FALSE) -> ()
          }
        }
        n84 = local read "stop"() -> (w175:bool)
      }
    }
  }
  n85 = VISA Close(VISA resource name=w3, error in (no error)=w2) -> ()  [unwired: 1 out]
